vi "SineGen IP.vi"(7 "Reset Accumulator":bool, 8 "Signal Offset":i16=-32768, 9 "Signal Amplitude (x 2^15)":u16=32768, 10 "Phase Shift":u32, 11 "Accumulator Increment":u32=100000) -> (2 "Accumulator":fxp<+,32,32>, 3 "Signal Value":i16)   [LabVIEW 2017, in "Oscillator.lvlib" / "Oscillator.lvclass"]
doc: "This VI generates the next point on a DDS generated sine wave.\n\nThe accumulator increments to calculate the next phase value in the waveform. By varying the accumulator increment you control the frequency of the sine wave.\n\nThe accumulator phase value is used to select a value from the sine wave reference waveform stored in the Lookup Table VI. The waveformcan be p[hase shifted by specifying a non-zero phase shift value which is added to the accumulator phase. The output from the LUT is scaled using the AO Amplitude value."
uses:
  Oscillator.lvclass
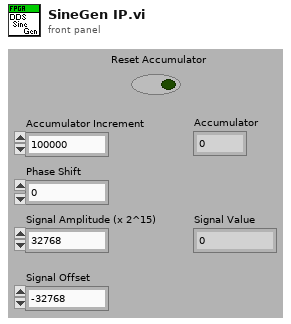
[diagram p1: front panel]
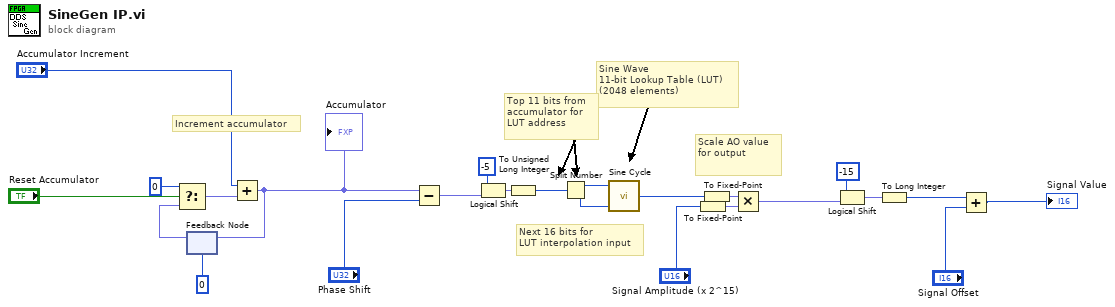
[diagram p0: block diagram]
diagram:
  # "Increment accumulator"
  # "Scale AO value\nfor output"
  # "Next 16 bits for\nLUT interpolation input"
  # "Top 11 bits from \naccumulator for\nLUT address"
  # "Sine Wave \n11-bit Lookup Table (LUT)\n(2048 elements)"
  n1 = feedback #1(u32 0) -> (w13:fxp<+,32,32>)
  n2 = Select(t=u32 0, s="Reset Accumulator", f=w13) -> (s? t:f=w14:fxp<+,32,32>)
  n3 = Add(x="Accumulator Increment", y=w14) -> (x+y=w11:fxp<+,32,32>)
  "Accumulator" <- w11
  n4 = feedback-in #1(w11) -> ()
  n5 = Subtract(x=w11, y="Phase Shift") -> (x-y=w18:fxp<+,32,32>)
  n6 = Logical Shift(y=-5, x=w18) -> (x << y=w23:fxp<+,32,32>)
  n7 = To Unsigned Long Integer(number=w23) -> (unsigned 32bit integer=w10:u32)
  n8 = Split Number(x=w10) -> (hi(x)=w24:u16, lo(x)=w7:u16)
  n9 = call "Sine Cycle"("address"=w24, "fractional index (x 2^16)"=w7) -> ("data out"=w6:i16)  [unwired: 7 in]
  n10 = To Fixed-Point(number="Signal Amplitude (x 2^15)") -> (fixed-point=w8:fxp<+,15,15>)  [unwired: 1 in]
  n11 = To Fixed-Point(number=w6) -> (fixed-point=w20:fxp<+/-,16,16>)  [unwired: 1 in]
  n12 = Multiply(x=w20, y=w8) -> (x*y=w4:fxp<+/-,32,32>)
  n13 = Logical Shift(y=-15, x=w4) -> (x << y=w3:fxp<+/-,32,32>)
  n14 = To Long Integer(number=w3) -> (32bit integer=w2:i32)
  n15 = Add(x=w2, y="Signal Offset") -> (x+y=→"Signal Value":i32)
